vi "Zero_Wheel_Find.vi"(2 "Limit":bool, 3 "Accum_Value":dbl, 4 "Reinit":bool) -> (0 "Wheel_Out":dbl, 1 "Zeroed?":bool)   [LabVIEW 2018]
uses:
  Zero_Wheels_Execute_Typedef.ctl
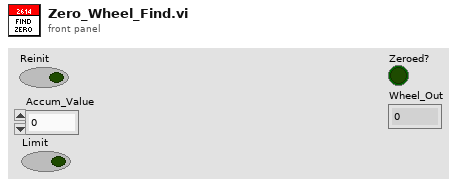
[diagram p1: front panel]
types:
  T1 = typedef "Zero_Wheels_Execute_Typedef.ctl" = enum16{"Wait_For_Press", "On_Zero_Spin", "Spin_to_Limit", "Write_Zero_Calculations"}
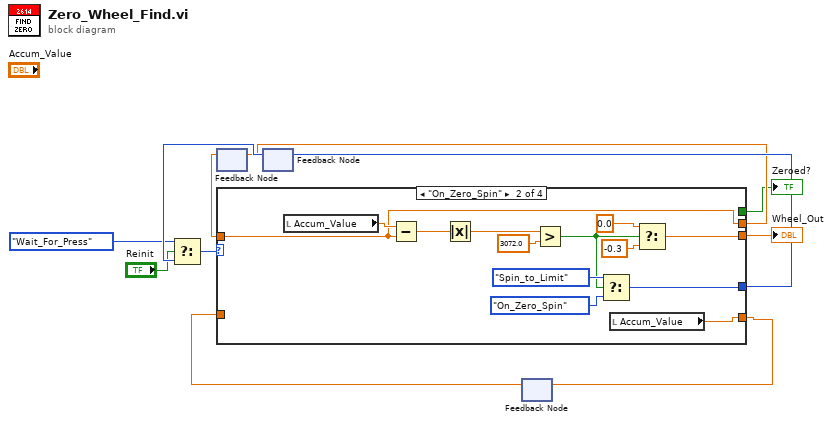
[diagram p0: block diagram]
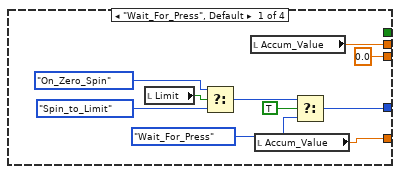
[diagram p2: hidden frame]
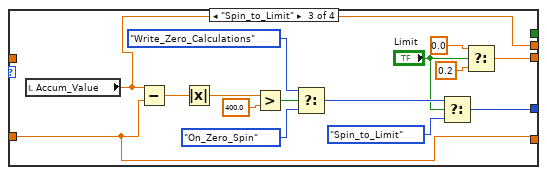
[diagram p3: hidden frame]
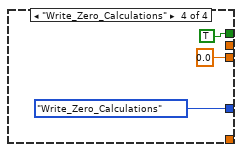
[diagram p4: hidden frame]
diagram:
  n1 = feedback #1() -> (w6:dbl)  [unwired: 1 in]
  n2 = feedback #2() -> (w10:T1)  [unwired: 1 in]
  n3 = Select(t=Zero_Wheels_Execute_Typedef."Wait_For_Press", s="Reinit", f=w10) -> (s? t:f=w8:T1)
  n4 = feedback #3() -> (w1:dbl)  [unwired: 1 in]
  n5 = case shown="\"On_Zero_Spin\"" w8 {
    tunnel: [w20 w28 w46 Zero_Wheels_Execute_Typedef."Write_Zero_Calculations" ("t")] -> w11
    tunnel: [0.0 ("f") w29 w47 0.0 ("f")] -> w3
    tunnel: w6 -> [_ w23 _ _]
    tunnel: [w13 w23 w35 _] -> w7
    tunnel: [_ _ _ TRUE ("Zero_Back_Left")] -> w4
    tunnel: [w12 w22 w36 _] -> w2
    tunnel: w1 -> [_ _ w36 _]
    frame "Wait_For_Press", Default {
      n6 = local read "Limit"() -> (w14:bool)
      n7 = Select(t=Zero_Wheels_Execute_Typedef."On_Zero_Spin", s=w14, f=Zero_Wheels_Execute_Typedef."Spin_to_Limit") -> (s? t:f=w19:T1)
      n8 = local read "Accum_Value"() -> (w13:dbl)
      n9 = local read "Accum_Value"() -> (w12:dbl)
      n10 = Select(t=w19, s=TRUE, f=Zero_Wheels_Execute_Typedef."Wait_For_Press") -> (s? t:f=w20:T1)
    }
    frame "On_Zero_Spin" {
      n11 = local read "Accum_Value"() -> (w24:dbl)
      n12 = Subtract(x=w24, y=w23) -> (x-y=w34:dbl)
      n13 = Absolute Value(x=w34) -> (abs(x)=w33:dbl)
      n14 = Greater?(x=w33, y=3072.0) -> (0:w25:bool)
      n15 = Select(t=Zero_Wheels_Execute_Typedef."Spin_to_Limit", s=w25, f=Zero_Wheels_Execute_Typedef."On_Zero_Spin" ("t")) -> (s? t:f=w28:T1)
      n16 = local read "Accum_Value"() -> (w22:dbl)
      n17 = Select(t=0.0, s=w25, f=-0.3) -> (s? t:f=w29:dbl)
    }
    frame "Spin_to_Limit" {
      n18 = local read "Accum_Value"() -> (w35:dbl)
      n19 = Subtract(x=w35, y=w36) -> (x-y=w45:dbl)
      n20 = Absolute Value(x=w45) -> (abs(x)=w44:dbl)
      n21 = Greater?(x=w44, y=400.0) -> (0:w38:bool)
      n22 = Select(t=Zero_Wheels_Execute_Typedef."Write_Zero_Calculations", s=w38, f=Zero_Wheels_Execute_Typedef."On_Zero_Spin" ("t")) -> (s? t:f=w42:T1)
      n23 = Select(t=w42, s="Limit", f=Zero_Wheels_Execute_Typedef."Spin_to_Limit" ("t")) -> (s? t:f=w46:T1)
      n24 = Select(t=0.0, s="Limit", f=0.2) -> (s? t:f=w47:dbl)
    }
    frame "Write_Zero_Calculations" {
    }
  }
  "Zeroed?" <- w4
  "Wheel_Out" <- w3
  n25 = feedback-in #1(w7) -> ()
  n26 = feedback-in #2(w11) -> ()
  n27 = feedback-in #3(w2) -> ()
